vi "Configure Charge Measurement Range Group.vi"(8 "error in (no error)":errorcluster, 10 "Range Group (0: HIGH)":i32(ring) items=["HIGH", "LOW"], 11 "VISA resource name":refnum<visa-resource-name>) -> (0 "error out":errorcluster, 3 "VISA resource name out":refnum<visa-resource-name>)   [LabVIEW 2016, in "Keithley 6517.lvlib"]
doc: "Configures the range group for the automatic measurement ranging operation at charge measurement."
uses:
  <instrlib>/Keithley 6517/Keithley 6517.lvlib
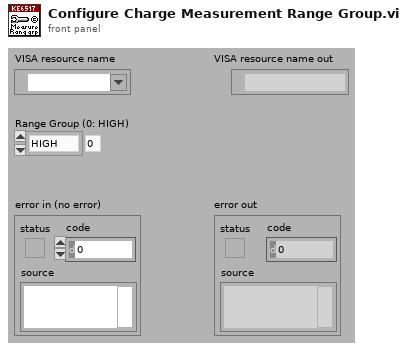
[diagram p1: front panel]
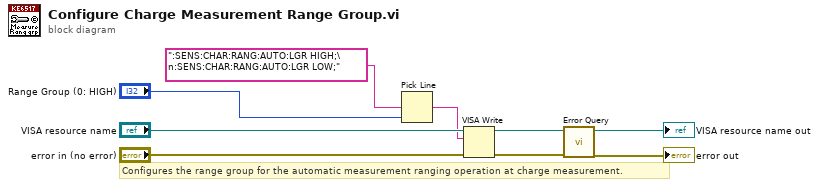
[diagram p0: block diagram]
diagram:
  # "Configures the range group for the automatic measurement ranging operation at charge measurement."
  n1 = Pick Line(multi-line string=":SENS:CHAR:RANG:AUTO:LGR HIGH;\n:SENS:CHAR:RANG:AUTO:LGR LOW;", line index="Range Group (0: HIGH)") -> (output string=w1:string)  [unwired: 1 in]
  n2 = VISA Write(VISA resource name="VISA resource name", write buffer=w1, error in (no error)="error in (no error)") -> (VISA resource name out=w7:refnum<visa-resource-name>, error out=w6:errorcluster)  [unwired: 1 out]
  n3 = call <instrlib>:"Error Query.vi"("error in (no error)"=w6, "VISA resource name"=w7) -> ("error out"=→"error out":errorcluster, "VISA resource name out"=→"VISA resource name out":refnum<visa-resource-name>)  [unwired: 6 in, 2 out]
